vi "App - analyze RUS V6.vi"() -> ()   [LabVIEW 2018] (continued)
ry\\September_2014\\091614\\91.68500K_500_2500_2.10000V_0.00000T_Sep16-2014__23-15-32_001_091614.bin", "mod time(min)"=58229475.53333333, "file format"=enum."binary", "power(V)"=2.1, "Magn Field(T) "=0.0}, {"temperature"=91.557, "temperature str"="91.55700", "file path"=path "D:/Data/Ultrasound/LSCO/LSCO22__130814c/5_Cooling_2nd_try/September_2014/091614/91.55700K_500_2500_2.10000V_0.00000T_Sep16-2014__23-16-52_001_091614.bin", "last mod"=timestamp(3493768612 s since 1904-01-01), "file name str"="D:\\Data\\Ultrasound\\LSCO\\LSCO22__130814c\\5_Cooling_2nd_try\\September_2014\\091614\\91.55700K_500_2500_2.10000V_0.00000T_Sep16-2014__23-16-52_001_091614.bin", "mod time(min)"=58229476.86666667, "file format"=enum."binary", "power(V)"=2.1, "Magn Field(T) "=0.0}, {"temperature"=91.423, "temperature str"="91.42300", "file path"=path "D:/Data/Ultrasound/LSCO/LSCO22__130814c/5_Cooling_2nd_try/September_2014/091614/91.42300K_500_2500_2.10000V_0.00000T_Sep16-2014__23-18-11_001_091614.bin", "last mod"=timestamp(3493768691 s since 1904-01-01), "file name str"="D:\\Data\\Ultrasound\\LSCO\\LSCO22__130814c\\5_Cooling_2nd_try\\September_2014\\091614\\91.42300K_500_2500_2.10000V_0.00000T_Sep16-2014__23-18-11_001_091614.bin", "mod time(min)"=58229478.18333333, "file format"=enum."binary", "power(V)"=2.1, "Magn Field(T) "=0.0}, {"temperature"=91.291, "temperature str"="91.29100", "file path"=path "D:/Data/Ultrasound/LSCO/LSCO22__130814c/5_Cooling_2nd_try/September_2014/091614/91.29100K_500_2500_2.10000V_0.00000T_Sep16-2014__23-19-30_001_091614.bin", "last mod"=timestamp(3493768770 s since 1904-01-01), "file name str"="D:\\Data\\Ultrasound\\LSCO\\LSCO22__130814c\\5_Cooling_2nd_try\\September_2014\\091614\\91.29100K_500_2500_2.10000V_0.00000T_Sep16-2014__23-19-30_001_091614.bin", "mod time(min)"=58229479.5, "file format"=enum."binary", "power(V)"=2.1, "Magn Field(T) "=0.0}, {"temperature"=91.167, "temperature str"="91.16700", "file path"=path "D:/Data/Ultrasound/LSCO/LSCO22__130814c/5_Cooling_2nd_try/September_2014/091614/91.16700K_500_2500_2.10000V_0.00000T_Sep16-2014__23-20-50_001_091614.bin", "last mod"=timestamp(3493768850 s since 1904-01-01), "file name str"="D:\\Data\\Ultrasound\\LSCO\\LSCO22__130814c\\5_Cooling_2nd_try\\September_2014\\091614\\91.16700K_500_2500_2.10000V_0.00000T_Sep16-2014__23-20-50_001_091614.bin", "mod time(min)"=58229480.833333336, "file format"=enum."binary", "power(V)"=2.1, "Magn Field(T) "=0.0}, {"temperature"=91.035, "temperature str"="91.03500", "file path"=path "D:/Data/Ultrasound/LSCO/LSCO22__130814c/5_Cooling_2nd_try/September_2014/091614/91.03500K_500_2500_2.10000V_0.00000T_Sep16-2014__23-22-09_001_091614.bin", "last mod"=timestamp(3493768929 s since 1904-01-01), "file name str"="D:\\Data\\Ultrasound\\LSCO\\LSCO22__130814c\\5_Cooling_2nd_try\\September_2014\\091614\\91.03500K_500_2500_2.10000V_0.00000T_Sep16-2014__23-22-09_001_091614.bin", "mod time(min)"=58229482.15, "file format"=enum."binary", "power(V)"=2.1, "Magn Field(T) "=0.0}, {"temperature"=90.91, "temperature str"="90.91000", "file path"=path "D:/Data/Ultrasound/LSCO/LSCO22__130814c/5_Cooling_2nd_try/September_2014/091614/90.91000K_500_2500_2.10000V_0.00000T_Sep16-2014__23-23-28_001_091614.bin", "last mod"=timestamp(3493769008 s since 1904-01-01), "file name str"="D:\\Data\\Ultrasound\\LSCO\\LSCO22__130814c\\5_Cooling_2nd_try\\September_2014\\091614\\90.91000K_500_2500_2.10000V_0.00000T_Sep16-2014__23-23-28_001_091614.bin", "mod time(min)"=58229483.46666667, "file format"=enum."binary", "power(V)"=2.1, "Magn Field(T) "=0.0}, {"temperature"=90.778, "temperature str"="90.77800", "file path"=path "D:/Data/Ultrasound/LSCO/LSCO22__130814c/5_Cooling_2nd_try/September_2014/091614/90.77800K_500_2500_2.10000V_0.00000T_Sep16-2014__23-24-48_001_091614.bin", "last mod"=timestamp(3493769088 s since 1904-01-01), "file name str"="D:\\Data\\Ultrasound\\LSCO\\LSCO22__130814c\\5_Cooling_2nd_try\\September_2014\\091614\\90.77800K_500_2500_2.10000V_0.00000T_Sep16-2014__23-24-48_001_091614.bin", "mod time(min)"=58229484.8, "file format"=enum."binary", "power(V)"=2.1, "Magn Field(T) "=0.0}, {"temperature"=90.65, "temperature str"="90.65000", "file path"=path "D:/Data/Ultrasound/LSCO/LSCO22__130814c/5_Cooling_2nd_try/September_2014/091614/90.65000K_500_2500_2.10000V_0.00000T_Sep16-2014__23-26-07_001_091614.bin", "last mod"=timestamp(3493769167 s since 1904-01-01), "file name str"="D:\\Data\\Ultrasound\\LSCO\\LSCO22__130814c\\5_Cooling_2nd_try\\September_2014\\091614\\90.65000K_500_2500_2.10000V_0.00000T_Sep16-2014__23-26-07_001_091614.bin", "mod time(min)"=58229486.11666667, "file format"=enum."binary", "power(V)"=2.1, "Magn Field(T) "=0.0}, {"temperature"=90.526, "temperature str"="90.52600", "file path"=path "D:/Data/Ultrasound/LSCO/LSCO22__130814c/5_Cooling_2nd_try/September_2014/091614/90.52600K_500_2500_2.10000V_0.00000T_Sep16-2014__23-27-26_001_091614.bin", "last mod"=timestamp(3493769246 s since 1904-01-01), "file name str"="D:\\Data\\Ultrasound\\LSCO\\LSCO22__130814c\\5_Cooling_2nd_try\\September_2014\\091614\\90.52600K_500_2500_2.10000V_0.00000T_Sep16-2014__23-27-26_001_091614.bin", "mod time(min)"=58229487.43333333, "file format"=enum."binary", "power(V)"=2.1, "Magn Field(T) "=0.0}, {"temperature"=90.397, "temperature str"="90.39700", "file path"=path "D:/Data/Ultrasound/LSCO/LSCO22__130814c/5_Cooling_2nd_try/September_2014/091614/90.39700K_500_2500_2.10000V_0.00000T_Sep16-2014__23-28-46_001_091614.bin", "last mod"=timestamp(3493769326 s since 1904-01-01), "file name str"="D:\\Data\\Ultrasound\\LSCO\\LSCO22__130814c\\5_Cooling_2nd_try\\September_2014\\091614\\90.39700K_500_2500_2.10000V_0.00000T_Sep16-2014__23-28-46_001_091614.bin", "mod time(min)"=58229488.766666666, "file format"=enum."binary", "power(V)"=2.1, "Magn Field(T) "=0.0}, {"temperature"=90.276, "temperature str"="90.27600", "file path"=path "D:/Data/Ultrasound/LSCO/LSCO22__130814c/5_Cooling_2nd_try/September_2014/091614/90.27600K_500_2500_2.10000V_0.00000T_Sep16-2014__23-30-05_001_091614.bin", "last mod"=timestamp(3493769405 s since 1904-01-01), "file name str"="D:\\Data\\Ultrasound\\LSCO\\LSCO22__130814c\\5_Cooling_2nd_try\\September_2014\\091614\\90.27600K_500_2500_2.10000V_0.00000T_Sep16-2014__23-30-05_001_091614.bin", "mod time(min)"=58229490.083333336, "file format"=enum."binary", "power(V)"=2.1, "Magn Field(T) "=0.0}, {"temperature"=90.146, "temperature str"="90.14600", "file path"=path "D:/Data/Ultrasound/LSCO/LSCO22__130814c/5_Cooling_2nd_try/September_2014/091614/90.14600K_500_2500_2.10000V_0.00000T_Sep16-2014__23-31-25_001_091614.bin", "last mod"=timestamp(3493769485 s since 1904-01-01), "file name str"="D:\\Data\\Ultrasound\\LSCO\\LSCO22__130814c\\5_Cooling_2nd_try\\September_2014\\091614\\90.14600K_500_2500_2.10000V_0.00000T_Sep16-2014__23-31-25_001_091614.bin", "mod time(min)"=58229491.416666664, "file format"=enum."binary", "power(V)"=2.1, "Magn Field(T) "=0.0}, {"temperature"=90.022, "temperature str"="90.02200", "file path"=path "D:/Data/Ultrasound/LSCO/LSCO22__130814c/5_Cooling_2nd_try/September_2014/091614/90.02200K_500_2500_2.10000V_0.00000T_Sep16-2014__23-32-44_001_091614.bin", "last mod"=timestamp(3493769564 s since 1904-01-01), "file name str"="D:\\Data\\Ultrasound\\LSCO\\LSCO22__130814c\\5_Cooling_2nd_try\\September_2014\\091614\\90.02200K_500_2500_2.10000V_0.00000T_Sep16-2014__23-32-44_001_091614.bin", "mod time(min)"=58229492.733333334, "file format"=enum."binary", "power(V)"=2.1, "Magn Field(T) "=0.0}, {"temperature"=89.9, "temperature str"="89.90000", "file path"=path "D:/Data/Ultrasound/LSCO/LSCO22__130814c/5_Cooling_2nd_try/September_2014/091614/89.90000K_500_2500_2.10000V_0.00000T_Sep16-2014__23-34-03_001_091614.bin", "last mod"=timestamp(3493769643 s since 1904-01-01), "file name str"="D:\\Data\\Ultrasound\\LSCO\\LSCO22__130814c\\5_Cooling_2nd_try\\September_2014\\091614\\89.90000K_500_2500_2.10000V_0.00000T_Sep16-2014__23-34-03_001_091614.bin", "mod time(min)"=58229494.05, "file format"=enum."binary", "power(V)"=2.1, "Magn Field(T) "=0.0}, {"temperature"=89.775, "temperature str"="89.77500", "file path"=path "D:/Data/Ultrasound/LSCO/LSCO22__130814c/5_Cooling_2nd_try/September_2014/091614/89.77500K_500_2500_2.10000V_0.00000T_Sep16-2014__23-35-23_001_091614.bin", "last mod"=timestamp(3493769723 s since 1904-01-01), "file name str"="D:\\Data\\Ultrasound\\LSCO\\LSCO22__130814c\\5_Cooling_2nd_try\\September_2014\\091614\\89.77500K_500_2500_2.10000V_0.00000T_Sep16-2014__23-35-23_001_091614.bin", "mod time(min)"=58229495.38333333, "file format"=enum."binary", "power(V)"=2.1, "Magn Field(T) "=0.0}, {"temperature"=89.652, "temperature str"="89.65200", "file path"=path "D:/Data/Ultrasound/LSCO/LSCO22__130814c/5_Cooling_2nd_try/September_2014/091614/89.65200K_500_2500_2.10000V_0.00000T_Sep16-2014__23-36-42_001_091614.bin", "last mod"=timestamp(3493769802 s since 1904-01-01), "file name str"="D:\\Data\\Ultrasound\\LSCO\\LSCO22__130814c\\5_Cooling_2nd_try\\September_2014\\091614\\89.65200K_500_2500_2.10000V_0.00000T_Sep16-2014__23-36-42_001_091614.bin", "mod time(min)"=58229496.7, "file format"=enum."binary", "power(V)"=2.1, "Magn Field(T) "=0.0}, {"temperature"=89.531, "temperature str"="89.53100", "file path"=path "D:/Data/Ultrasound/LSCO/LSCO22__130814c/5_Cooling_2nd_try/September_2014/091614/89.53100K_500_2500_2.10000V_0.00000T_Sep16-2014__23-38-01_001_091614.bin", "last mod"=timestamp(3493769881 s since 1904-01-01), "file name str"="D:\\Data\\Ultrasound\\LSCO\\LSCO22__130814c\\5_Cooling_2nd_try\\September_2014\\091614\\89.53100K_500_2500_2.10000V_0.00000T_Sep16-2014__23-38-01_001_091614.bin", "mod time(min)"=58229498.016666666, "file format"=enum."binary", "power(V)"=2.1, "Magn Field(T) "=0.0}, {"temperature"=89.405, "temperature str"="89.40500", "file path"=path "D:/Data/Ultrasound/LSCO/LSCO22__130814c/5_Cooling_2nd_try/September_2014/091614/89.40500K_500_2500_2.10000V_0.00000T_Sep16-2014__23-39-21_001_091614.bin", "last mod"=timestamp(3493769961 s since 1904-01-01), "file name str"="D:\\Data\\Ultrasound\\LSCO\\LSCO22__130814c\\5_Cooling_2nd_try\\September_2014\\091614\\89.40500K_500_2500_2.10000V_0.00000T_Sep16-2014__23-39-21_001_091614.bin", "mod time(min)"=58229499.35, "file format"=enum."binary", "power(V)"=2.1, "Magn Field(T) "=0.0}, {"temperature"=89.288, "temperature str"="89.28800", "file path"=path "D:/Data/Ultrasound/LSCO/LSCO22__130814c/5_Cooling_2nd_try/September_2014/091614/89.28800K_500_2500_2.10000V_0.00000T_Sep16-2014__23-40-40_001_091614.bin", "last mod"=timestamp(3493770040 s since 1904-01-01), "file name str"="D:\\Data\\Ultrasound\\LSCO\\LSCO22__130814c\\5_Cooling_2nd_try\\September_2014\\091614\\89.28800K_500_2500_2.10000V_0.00000T_Sep16-2014__23-40-40_001_091614.bin", "mod time(min)"=58229500.666666664, "file format"=enum."binary", "power(V)"=2.1, "Magn Field(T) "=0.0}, {"temperature"=89.165, "temperature str"="89.16500", "file path"=path "D:/Data/Ultrasound/LSCO/LSCO22__130814c/5_Cooling_2nd_try/September_2014/091614/89.16500K_500_2500_2.10000V_0.00000T_Sep16-2014__23-42-00_001_091614.bin", "last mod"=timestamp(3493770120 s since 1904-01-01), "file name str"="D:\\Data\\Ultrasound\\LSCO\\LSCO22__130814c\\5_Cooling_2nd_try\\September_2014\\091614\\89.16500K_500_2500_2.10000V_0.00000T_Sep16-2014__23-42-00_001_091614.bin", "mod time(min)"=58229502.0, "file format"=enum."binary", "power(V)"=2.1, "Magn Field(T) "=0.0}, {"temperature"=89.042, "temperature str"="89.04200", "file path"=path "D:/Data/Ultrasound/LSCO/LSCO22__130814c/5_Cooling_2nd_try/September_2014/091614/89.04200K_500_2500_2.10000V_0.00000T_Sep16-2014__23-43-19_001_091614.bin", "last mod"=timestamp(3493770199 s since 1904-01-01), "file name str"="D:\\Data\\Ultrasound\\LSCO\\LSCO22__130814c\\5_Cooling_2nd_try\\September_2014\\091614\\89.04200K_500_2500_2.10000V_0.00000T_Sep16-2014__23-43-19_001_091614.bin", "mod time(min)"=58229503.31666667, "file format"=enum."binary", "power(V)"=2.1, "Magn Field(T) "=0.0}, {"temperature"=88.925, "temperature str"="88.92500", "file path"=path "D:/Data/Ultrasound/LSCO/LSCO22__130814c/5_Cooling_2nd_try/September_2014/091614/88.92500K_500_2500_2.10000V_0.00000T_Sep16-2014__23-44-38_001_091614.bin", "last mod"=timestamp(3493770278 s since 1904-01-01), "file name str"="D:\\Data\\Ultrasound\\LSCO\\LSCO22__130814c\\5_Cooling_2nd_try\\September_2014\\091614\\88.92500K_500_2500_2.10000V_0.00000T_Sep16-2014__23-44-38_001_091614.bin", "mod time(min)"=58229504.63333333, "file format"=enum."binary", "power(V)"=2.1, "Magn Field(T) "=0.0}, {"temperature"=88.804, "temperature str"="88.80400", "file path"=path "D:/Data/Ultrasound/LSCO/LSCO22__130814c/5_Cooling_2nd_try/September_2014/091614/88.80400K_500_2500_2.10000V_0.00000T_Sep16-2014__23-45-58_001_091614.bin", "last mod"=timestamp(3493770358 s since 1904-01-01), "file name str"="D:\\Data\\Ultrasound\\LSCO\\LSCO22__130814c\\5_Cooling_2nd_try\\September_2014\\091614\\88.80400K_500_2500_2.10000V_0.00000T_Sep16-2014__23-45-58_001_091614.bin", "mod time(min)"=58229505.96666667, "file format"=enum."binary", "power(V)"=2.1, "Magn Field(T) "=0.0}, {"temperature"=88.687, "temperature str"="88.68700", "file path"=path "D:/Data/Ultrasound/LSCO/LSCO22__130814c/5_Cooling_2nd_try/September_2014/091614/88.68700K_500_2500_2.10000V_0.00000T_Sep16-2014__23-47-17_001_091614.bin", "last mod"=timestamp(3493770437 s since 1904-01-01), "file name str"="D:\\Data\\Ultrasound\\LSCO\\LSCO22__130814c\\5_Cooling_2nd_try\\September_2014\\091614\\88.68700K_500_2500_2.10000V_0.00000T_Sep16-2014__23-47-17_001_091614.bin", "mod time(min)"=58229507.28333333, "file format"=enum."binary", "power(V)"=2.1, "Magn Field(T) "=0.0}, {"temperature"=88.566, "temperature str"="88.56600", "file path"=path "D:/Data/Ultrasound/LSCO/LSCO22__130814c/5_Cooling_2nd_try/September_2014/091614/88.56600K_500_2500_2.10000V_0.00000T_Sep16-2014__23-48-36_001_091614.bin", "last mod"=timestamp(3493770516 s since 1904-01-01), "file name str"="D:\\Data\\Ultrasound\\LSCO\\LSCO22__130814c\\5_Cooling_2nd_try\\September_2014\\091614\\88.56600K_500_2500_2.10000V_0.00000T_Sep16-2014__23-48-36_001_091614.bin", "mod time(min)"=58229508.6, "file format"=enum."binary", "power(V)"=2.1, "Magn Field(T) "=0.0}, {"temperature"=88.447, "temperature str"="88.44700", "file path"=path "D:/Data/Ultrasound/LSCO/LSCO22__130814c/5_Cooling_2nd_try/September_2014/091614/88.44700K_500_2500_2.10000V_0.00000T_Sep16-2014__23-49-56_001_091614.bin", "last mod"=timestamp(3493770596 s since 1904-01-01), "file name str"="D:\\Data\\Ultrasound\\LSCO\\LSCO22__130814c\\5_Cooling_2nd_try\\September_2014\\091614\\88.44700K_500_2500_2.10000V_0.00000T_Sep16-2014__23-49-56_001_091614.bin", "mod time(min)"=58229509.93333333, "file format"=enum."binary", "power(V)"=2.1, "Magn Field(T) "=0.0}, {"temperature"=88.332, "temperature str"="88.33200", "file path"=path "D:/Data/Ultrasound/LSCO/LSCO22__130814c/5_Cooling_2nd_try/September_2014/091614/88.33200K_500_2500_2.10000V_0.00000T_Sep16-2014__23-51-15_001_091614.bin", "last mod"=timestamp(3493770675 s since 1904-01-01), "file name str"="D:\\Data\\Ultrasound\\LSCO\\LSCO22__130814c\\5_Cooling_2nd_try\\September_2014\\091614\\88.33200K_500_2500_2.10000V_0.00000T_Sep16-2014__23-51-15_001_091614.bin", "mod time(min)"=58229511.25, "file format"=enum."binary", "power(V)"=2.1, "Magn Field(T) "=0.0}, {"temperature"=88.213, "temperature str"="88.21300", "file path"=path "D:/Data/Ultrasound/LSCO/LSCO22__130814c/5_Cooling_2nd_try/September_2014/091614/88.21300K_500_2500_2.10000V_0.00000T_Sep16-2014__23-52-35_001_091614.bin", "last mod"=timestamp(3493770755 s since 1904-01-01), "file name str"="D:\\Data\\Ultrasound\\LSCO\\LSCO22__130814c\\5_Cooling_2nd_try\\September_2014\\091614\\88.21300K_500_2500_2.10000V_0.00000T_Sep16-2014__23-52-35_001_091614.bin", "mod time(min)"=58229512.583333336, "file format"=enum."binary", "power(V)"=2.1, "Magn Field(T) "=0.0}, {"temperature"=88.1, "temperature str"="88.10000", "file path"=path "D:/Data/Ultrasound/LSCO/LSCO22__130814c/5_Cooling_2nd_try/September_2014/091614/88.10000K_500_2500_2.10000V_0.00000T_Sep16-2014__23-53-54_001_091614.bin", "last mod"=timestamp(3493770834 s since 1904-01-01), "file name str"="D:\\Data\\Ultrasound\\LSCO\\LSCO22__130814c\\5_Cooling_2nd_try\\September_2014\\091614\\88.10000K_500_2500_2.10000V_0.00000T_Sep16-2014__23-53-54_001_091614.bin", "mod time(min)"=58229513.9, "file format"=enum."binary", "power(V)"=2.1, "Magn Field(T) "=0.0}, {"temperature"=87.983, "temperature str"="87.98300", "file path"=path "D:/Data/Ultrasound/LSCO/LSCO22__130814c/5_Cooling_2nd_try/September_2014/091614/87.98300K_500_2500_2.10000V_0.00000T_Sep16-2014__23-55-13_001_091614.bin", "last mod"=timestamp(3493770913 s since 1904-01-01), "file name str"="D:\\Data\\Ultrasound\\LSCO\\LSCO22__130814c\\5_Cooling_2nd_try\\September_2014\\091614\\87.98300K_500_2500_2.10000V_0.00000T_Sep16-2014__23-55-13_001_091614.bin", "mod time(min)"=58229515.21666667, "file format"=enum."binary", "power(V)"=2.1, "Magn Field(T) "=0.0}, {"temperature"=87.861, "temperature str"="87.86100", "file path"=path "D:/Data/Ultrasound/LSCO/LSCO22__130814c/5_Cooling_2nd_try/September_2014/091614/87.86100K_500_2500_2.10000V_0.00000T_Sep16-2014__23-56-33_001_091614.bin", "last mod"=timestamp(3493770993 s since 1904-01-01), "file name str"="D:\\Data\\Ultrasound\\LSCO\\LSCO22__130814c\\5_Cooling_2nd_try\\September_2014\\091614\\87.86100K_500_2500_2.10000V_0.00000T_Sep16-2014__23-56-33_001_091614.bin", "mod time(min)"=58229516.55, "file format"=enum."binary", "power(V)"=2.1, "Magn Field(T) "=0.0}, {"temperature"=87.751, "temperature str"="87.75100", "file path"=path "D:/Data/Ultrasound/LSCO/LSCO22__130814c/5_Cooling_2nd_try/September_2014/091614/87.75100K_500_2500_2.10000V_0.00000T_Sep16-2014__23-57-52_001_091614.bin", "last mod"=timestamp(3493771072 s since 1904-01-01), "file name str"="D:\\Data\\Ultrasound\\LSCO\\LSCO22__130814c\\5_Cooling_2nd_try\\September_2014\\091614\\87.75100K_500_2500_2.10000V_0.00000T_Sep16-2014__23-57-52_001_091614.bin", "mod time(min)"=58229517.86666667, "file format"=enum."binary", "power(V)"=2.1, "Magn Field(T) "=0.0}, {"temperature"=87.635, "temperature str"="87.63500", "file path"=path "D:/Data/Ultrasound/LSCO/LSCO22__130814c/5_Cooling_2nd_try/September_2014/091714/87.63500K_500_2500_2.10000V_0.00000T_Sep16-2014__23-59-11_001_091714.bin", "last mod"=timestamp(3493771151 s since 1904-01-01), "file name str"="D:\\Data\\Ultrasound\\LSCO\\LSCO22__130814c\\5_Cooling_2nd_try\\September_2014\\091714\\87.63500K_500_2500_2.10000V_0.00000T_Sep16-2014__23-59-11_001_091714.bin", "mod time(min)"=58229519.18333333, "file format"=enum."binary", "power(V)"=2.1, "Magn Field(T) "=0.0}, {"temperature"=87.523, "temperature str"="87.52300", "file path"=path "D:/Data/Ultrasound/LSCO/LSCO22__130814c/5_Cooling_2nd_try/September_2014/091714/87.52300K_500_2500_2.10000V_0.00000T_Sep17-2014__00-00-31_001_091714.bin", "last mod"=timestamp(3493771231 s since 1904-01-01), "file name str"="D:\\Data\\Ultrasound\\LSCO\\LSCO22__130814c\\5_Cooling_2nd_try\\September_2014\\091714\\87.52300K_500_2500_2.10000V_0.00000T_Sep17-2014__00-00-31_001_091714.bin", "mod time(min)"=58229520.516666666, "file format"=enum."binary", "power(V)"=2.1, "Magn Field(T) "=0.0}, {"temperature"=87.407, "temperature str"="87.40700", "file path"=path "D:/Data/Ultrasound/LSCO/LSCO22__130814c/5_Cooling_2nd_try/September_2014/091714/87.40700K_500_2500_2.10000V_0.00000T_Sep17-2014__00-01-50_001_091714.bin", "last mod"=timestamp(3493771310 s since 1904-01-01), "file name str"="D:\\Data\\Ultrasound\\LSCO\\LSCO22__130814c\\5_Cooling_2nd_try\\September_2014\\091714\\87.40700K_500_2500_2.10000V_0.00000T_Sep17-2014__00-01-50_001_091714.bin", "mod time(min)"=58229521.833333336, "file format"=enum."binary", "power(V)"=2.1, "Magn Field(T) "=0.0}, {"temperature"=87.293, "temperature str"="87.29300", "file path"=path "D:/Data/Ultrasound/LSCO/LSCO22__130814c/5_Cooling_2nd_try/September_2014/091714/87.29300K_500_2500_2.10000V_0.00000T_Sep17-2014__00-03-10_001_091714.bin", "last mod"=timestamp(3493771390 s since 1904-01-01), "file name str"="D:\\Data\\Ultrasound\\LSCO\\LSCO22__130814c\\5_Cooling_2nd_try\\September_2014\\091714\\87.29300K_500_2500_2.10000V_0.00000T_Sep17-2014__00-03-10_001_091714.bin", "mod time(min)"=58229523.166666664, "file format"=enum."binary", "power(V)"=2.1, "Magn Field(T) "=0.0}, {"temperature"=87.182, "temperature str"="87.18200", "file path"=path "D:/Data/Ultrasound/LSCO/LSCO22__130814c/5_Cooling_2nd_try/September_2014/091714/87.18200K_500_2500_2.10000V_0.00000T_Sep17-2014__00-04-29_001_091714.bin", "last mod"=timestamp(3493771469 s since 1904-01-01), "file name str"="D:\\Data\\Ultrasound\\LSCO\\LSCO22__130814c\\5_Cooling_2nd_try\\September_2014\\091714\\87.18200K_500_2500_2.10000V_0.00000T_Sep17-2014__00-04-29_001_091714.bin", "mod time(min)"=58229524.483333334, "file format"=enum."binary", "power(V)"=2.1, "Magn Field(T) "=0.0}, {"temperature"=87.068, "temperature str"="87.06800", "file path"=path "D:/Data/Ultrasound/LSCO/LSCO22__130814c/5_Cooling_2nd_try/September_2014/091714/87.06800K_500_2500_2.10000V_0.00000T_Sep17-2014__00-05-48_001_091714.bin", "last mod"=timestamp(3493771548 s since 1904-01-01), "file name str"="D:\\Data\\Ultrasound\\LSCO\\LSCO22__130814c\\5_Cooling_2nd_try\\September_2014\\091714\\87.06800K_500_2500_2.10000V_0.00000T_Sep17-2014__00-05-48_001_091714.bin", "mod time(min)"=58229525.8, "file format"=enum."binary", "power(V)"=2.1, "Magn Field(T) "=0.0}, {"temperature"=86.958, "temperature str"="86.95800", "file path"=path "D:/Data/Ultrasound/LSCO/LSCO22__130814c/5_Cooling_2nd_try/September_2014/091714/86.95800K_500_2500_2.10000V_0.00000T_Sep17-2014__00-07-08_001_091714.bin", "last mod"=timestamp(3493771628 s since 1904-01-01), "file name str"="D:\\Data\\Ultrasound\\LSCO\\LSCO22__130814c\\5_Cooling_2nd_try\\September_2014\\091714\\86.95800K_500_2500_2.10000V_0.00000T_Sep17-2014__00-07-08_001_091714.bin", "mod time(min)"=58229527.13333333, "file format"=enum."binary", "power(V)"=2.1, "Magn Field(T) "=0.0}, {"temperature"=86.845, "temperature str"="86.84500", "file path"=path "D:/Data/Ultrasound/LSCO/LSCO22__130814c/5_Cooling_2nd_try/September_2014/091714/86.84500K_500_2500_2.10000V_0.00000T_Sep17-2014__00-08-27_001_091714.bin", "last mod"=timestamp(3493771707 s since 1904-01-01), "file name str"="D:\\Data\\Ultrasound\\LSCO\\LSCO22__130814c\\5_Cooling_2nd_try\\September_2014\\091714\\86.84500K_500_2500_2.10000V_0.00000T_Sep17-2014__00-08-27_001_091714.bin", "mod time(min)"=58229528.45, "file format"=enum."binary", "power(V)"=2.1, "Magn Field(T) "=0.0}, {"temperature"=86.732, "temperature str"="86.73200", "file path"=path "D:/Data/Ultrasound/LSCO/LSCO22__130814c/5_Cooling_2nd_try/September_2014/091714/86.73200K_500_2500_2.10000V_0.00000T_Sep17-2014__00-09-46_001_091714.bin", "last mod"=timestamp(3493771786 s since 1904-01-01), "file name str"="D:\\Data\\Ultrasound\\LSCO\\LSCO22__130814c\\5_Cooling_2nd_try\\September_2014\\091714\\86.73200K_500_2500_2.10000V_0.00000T_Sep17-2014__00-09-46_001_091714.bin", "mod time(min)"=58229529.766666666, "file format"=enum."binary", "power(V)"=2.1, "Magn Field(T) "=0.0}, {"temperature"=86.623, "temperature str"="86.62300", "file path"=path "D:/Data/Ultrasound/LSCO/LSCO22__130814c/5_Cooling_2nd_try/September_2014/091714/86.62300K_500_2500_2.10000V_0.00000T_Sep17-2014__00-11-06_001_091714.bin", "last mod"=timestamp(3493771866 s since 1904-01-01), "file name str"="D:\\Data\\Ultrasound\\LSCO\\LSCO22__130814c\\5_Cooling_2nd_try\\September_2014\\091714\\86.62300K_500_2500_2.10000V_0.00000T_Sep17-2014__00-11-06_001_091714.bin", "mod time(min)"=58229531.1, "file format"=enum."binary", "power(V)"=2.1, "Magn Field(T) "=0.0}, {"temperature"=86.512, "temperature str"="86.51200", "file path"=path "D:/Data/Ultrasound/LSCO/LSCO22__130814c/5_Cooling_2nd_try/September_2014/091714/86.51200K_500_2500_2.10000V_0.00000T_Sep17-2014__00-12-25_001_091714.bin", "last mod"=timestamp(3493771945 s since 1904-01-01), "file name str"="D:\\Data\\Ultrasound\\LSCO\\LSCO22__130814c\\5_Cooling_2nd_try\\September_2014\\091714\\86.51200K_500_2500_2.10000V_0.00000T_Sep17-2014__00-12-25_001_091714.bin", "mod time(min)"=58229532.416666664, "file format"=enum."binary", "power(V)"=2.1, "Magn Field(T) "=0.0}, {"temperature"=86.405, "temperature str"="86.40500", "file path"=path "D:/Data/Ultrasound/LSCO/LSCO22__130814c/5_Cooling_2nd_try/September_2014/091714/86.40500K_500_2500_2.10000V_0.00000T_Sep17-2014__00-13-45_001_091714.bin", "last mod"=timestamp(3493772025 s since 1904-01-01), "file name str"="D:\\Data\\Ultrasound\\LSCO\\LSCO22__130814c\\5_Cooling_2nd_try\\September_2014\\091714\\86.40500K_500_2500_2.10000V_0.00000T_Sep17-2014__00-13-45_001_091714.bin", "mod time(min)"=58229533.75, "file format"=enum."binary", "power(V)"=2.1, "Magn Field(T) "=0.0}, {"temperature"=86.294, "temperature str"="86.29400", "file path"=path "D:/Data/Ultrasound/LSCO/LSCO22__130814c/5_Cooling_2nd_try/September_2014/091714/86.29400K_500_2500_2.10000V_0.00000T_Sep17-2014__00-15-04_001_091714.bin", "last mod"=timestamp(3493772104 s since 1904-01-01), "file name str"="D:\\Data\\Ultrasound\\LSCO\\LSCO22__130814c\\5_Cooling_2nd_try\\September_2014\\091714\\86.29400K_500_2500_2.10000V_0.00000T_Sep17-2014__00-15-04_001_091714.bin", "mod time(min)"=58229535.06666667, "file format"=enum."binary", "power(V)"=2.1, "Magn Field(T) "=0.0}, {"temperature"=86.184, "temperature str"="86.18400", "file path"=path "D:/Data/Ultrasound/LSCO/LSCO22__130814c/5_Cooling_2nd_try/September_2014/091714/86.18400K_500_2500_2.10000V_0.00000T_Sep17-2014__00-16-23_001_091714.bin", "last mod"=timestamp(3493772183 s since 1904-01-01), "file name str"="D:\\Data\\Ultrasound\\LSCO\\LSCO22__130814c\\5_Cooling_2nd_try\\September_2014\\091714\\86.18400K_500_2500_2.10000V_0.00000T_Sep17-2014__00-16-23_001_091714.bin", "mod time(min)"=58229536.38333333, "file format"=enum."binary", "power(V)"=2.1, "Magn Field(T) "=0.0}, {"temperature"=86.077, "temperature str"="86.07700", "file path"=path "D:/Data/Ultrasound/LSCO/LSCO22__130814c/5_Cooling_2nd_try/September_2014/091714/86.07700K_500_2500_2.10000V_0.00000T_Sep17-2014__00-17-43_001_091714.bin", "last mod"=timestamp(3493772263 s since 1904-01-01), "file name str"="D:\\Data\\Ultrasound\\LSCO\\LSCO22__130814c\\5_Cooling_2nd_try\\September_2014\\091714\\86.07700K_500_2500_2.10000V_0.00000T_Sep17-2014__00-17-43_001_091714.bin", "mod time(min)"=58229537.71666667, "file format"=enum."binary", "power(V)"=2.1, "Magn Field(T) "=0.0}, {"temperature"=85.969, "temperature str"="85.96900", "file path"=path "D:/Data/Ultrasound/LSCO/LSCO22__130814c/5_Cooling_2nd_try/September_2014/091714/85.96900K_500_2500_2.10000V_0.00000T_Sep17-2014__00-19-02_001_091714.bin", "last mod"=timestamp(3493772342 s since 1904-01-01), "file name str"="D:\\Data\\Ultrasound\\LSCO\\LSCO22__130814c\\5_Cooling_2nd_try\\September_2014\\091714\\85.96900K_500_2500_2.10000V_0.00000T_Sep17-2014__00-19-02_001_091714.bin", "mod time(min)"=58229539.03333333, "file format"=enum."binary", "power(V)"=2.1, "Magn Field(T) "=0.0}, {"temperature"=85.861, "temperature str"="85.86100", "file path"=path "D:/Data/Ultrasound/LSCO/LSCO22__130814c/5_Cooling_2nd_try/September_2014/091714/85.86100K_500_2500_2.10000V_0.00000T_Sep17-2014__00-20-21_001_091714.bin", "last mod"=timestamp(3493772421 s since 1904-01-01), "file name str"="D:\\Data\\Ultrasound\\LSCO\\LSCO22__130814c\\5_Cooling_2nd_try\\September_2014\\091714\\85.86100K_500_2500_2.10000V_0.00000T_Sep17-2014__00-20-21_001_091714.bin", "mod time(min)"=58229540.35, "file format"=enum."binary", "power(V)"=2.1, "Magn Field(T) "=0.0}, {"temperature"=85.752, "temperature str"="85.75200", "file path"=path "D:/Data/Ultrasound/LSCO/LSCO22__130814c/5_Cooling_2nd_try/September_2014/091714/85.75200K_500_2500_2.10000V_0.00000T_Sep17-2014__00-21-41_001_091714.bin", "last mod"=timestamp(3493772501 s since 1904-01-01), "file name str"="D:\\Data\\Ultrasound\\LSCO\\LSCO22__130814c\\5_Cooling_2nd_try\\September_2014\\091714\\85.75200K_500_2500_2.10000V_0.00000T_Sep17-2014__00-21-41_001_091714.bin", "mod time(min)"=58229541.68333333, "file format"=enum."binary", "power(V)"=2.1, "Magn Field(T) "=0.0}, {"temperature"=85.645, "temperature str"="85.64500", "file path"=path "D:/Data/Ultrasound/LSCO/LSCO22__130814c/5_Cooling_2nd_try/September_2014/091714/85.64500K_500_2500_2.10000V_0.00000T_Sep17-2014__00-23-00_001_091714.bin", "last mod"=timestamp(3493772580 s since 1904-01-01), "file name str"="D:\\Data\\Ultrasound\\LSCO\\LSCO22__130814c\\5_Cooling_2nd_try\\September_2014\\091714\\85.64500K_500_2500_2.10000V_0.00000T_Sep17-2014__00-23-00_001_091714.bin", "mod time(min)"=58229543.0, "file format"=enum."binary", "power(V)"=2.1, "Magn Field(T) "=0.0}, {"temperature"=85.541, "temperature str"="85.54100", "file path"=path "D:/Data/Ultrasound/LSCO/LSCO22__130814c/5_Cooling_2nd_try/September_2014/091714/85.54100K_500_2500_2.10000V_0.00000T_Sep17-2014__00-24-20_001_091714.bin", "last mod"=timestamp(3493772660 s since 1904-01-01), "file name str"="D:\\Data\\Ultrasound\\LSCO\\LSCO22__130814c\\5_Cooling_2nd_try\\September_2014\\091714\\85.54100K_500_2500_2.10000V_0.00000T_Sep17-2014__00-24-20_001_091714.bin", "mod time(min)"=58229544.333333336, "file format"=enum."binary", "power(V)"=2.1, "Magn Field(T) "=0.0}, {"temperature"=85.433, "temperature str"="85.43300", "file path"=path "D:/Data/Ultrasound/LSCO/LSCO22__130814c/5_Cooling_2nd_try/September_2014/091714/85.43300K_500_2500_2.10000V_0.00000T_Sep17-2014__00-25-39_001_091714.bin", "last mod"=timestamp(3493772739 s since 1904-01-01), "file name str"="D:\\Data\\Ultrasound\\LSCO\\LSCO22__130814c\\5_Cooling_2nd_try\\September_2014\\091714\\85.43300K_500_2500_2.10000V_0.00000T_Sep17-2014__00-25-39_001_091714.bin", "mod time(min)"=58229545.65, "file format"=enum."binary", "power(V)"=2.1, "Magn Field(T) "=0.0}, {"temperature"=85.328, "temperature str"="85.32800", "file path"=path "D:/Data/Ultrasound/LSCO/LSCO22__130814c/5_Cooling_2nd_try/September_2014/091714/85.32800K_500_2500_2.10000V_0.00000T_Sep17-2014__00-26-58_001_091714.bin", "last mod"=timestamp(3493772818 s since 1904-01-01), "file name str"="D:\\Data\\Ultrasound\\LSCO\\LSCO22__130814c\\5_Cooling_2nd_try\\September_2014\\091714\\85.32800K_500_2500_2.10000V_0.00000T_Sep17-2014__00-26-58_001_091714.bin", "mod time(min)"=58229546.96666667, "file format"=enum."binary", "power(V)"=2.1, "Magn Field(T) "=0.0}, {"temperature"=85.224, "temperature str"="85.22400", "file path"=path "D:/Data/Ultrasound/LSCO/LSCO22__130814c/5_Cooling_2nd_try/September_2014/091714/85.22400K_500_2500_2.10000V_0.00000T_Sep17-2014__00-28-18_001_091714.bin", "last mod"=timestamp(3493772898 s since 1904-01-01), "file name str"="D:\\Data\\Ultrasound\\LSCO\\LSCO22__130814c\\5_Cooling_2nd_try\\September_2014\\091714\\85.22400K_500_2500_2.10000V_0.00000T_Sep17-2014__00-28-18_001_091714.bin", "mod time(min)"=58229548.3, "file format"=enum."binary", "power(V)"=2.1, "Magn Field(T) "=0.0}, {"temperature"=85.117, "temperature str"="85.11700", "file path"=path "D:/Data/Ultrasound/LSCO/LSCO22__130814c/5_Cooling_2nd_try/September_2014/091714/85.11700K_500_2500_2.10000V_0.00000T_Sep17-2014__00-29-37_001_091714.bin", "last mod"=timestamp(3493772977 s since 1904-01-01), "file name str"="D:\\Data\\Ultrasound\\LSCO\\LSCO22__130814c\\5_Cooling_2nd_try\\September_2014\\091714\\85.11700K_500_2500_2.10000V_0.00000T_Sep17-2014__00-29-37_001_091714.bin", "mod time(min)"=58229549.61666667, "file format"=enum."binary", "power(V)"=2.1, "Magn Field(T) "=0.0}, {"temperature"=85.014, "temperature str"="85.01400", "file path"=path "D:/Data/Ultrasound/LSCO/LSCO22__130814c/5_Cooling_2nd_try/September_2014/091714/85.01400K_500_2500_2.10000V_0.00000T_Sep17-2014__00-30-56_001_091714.bin", "last mod"=timestamp(3493773056 s since 1904-01-01), "file name str"="D:\\Data\\Ultrasound\\LSCO\\LSCO22__130814c\\5_Cooling_2nd_try\\September_2014\\091714\\85.01400K_500_2500_2.10000V_0.00000T_Sep17-2014__00-30-56_001_091714.bin", "mod time(min)"=58229550.93333333, "file format"=enum."binary", "power(V)"=2.1, "Magn Field(T) "=0.0}, {"temperature"=84.907, "temperature str"="84.90700", "file path"=path "D:/Data/Ultrasound/LSCO/LSCO22__130814c/5_Cooling_2nd_try/September_2014/091714/84.90700K_500_2500_2.10000V_0.00000T_Sep17-2014__00-32-16_001_091714.bin", "last mod"=timestamp(3493773136 s since 1904-01-01), "file name str"="D:\\Data\\Ultrasound\\LSCO\\LSCO22__130814c\\5_Cooling_2nd_try\\September_2014\\091714\\84.90700K_500_2500_2.10000V_0.00000T_Sep17-2014__00-32-16_001_091714.bin", "mod time(min)"=58229552.266666666, "file format"=enum."binary", "power(V)"=2.1, "Magn Field(T) "=0.0}, {"temperature"=84.805, "temperature str"="84.80500", "file path"=path "D:/Data/Ultrasound/LSCO/LSCO22__130814c/5_Cooling_2nd_try/September_2014/091714/84.80500K_500_2500_2.10000V_0.00000T_Sep17-2014__00-33-35_001_091714.bin", "last mod"=timestamp(3493773215 s since 1904-01-01), "file name str"="D:\\Data\\Ultrasound\\LSCO\\LSCO22__130814c\\5_Cooling_2nd_try\\September_2014\\091714\\84.80500K_500_2500_2.10000V_0.00000T_Sep17-2014__00-33-35_001_091714.bin", "mod time(min)"=58229553.583333336, "file format"=enum."binary", "power(V)"=2.1, "Magn Field(T) "=0.0}, {"temperature"=84.704, "temperature str"="84.70400", "file path"=path "D:/Data/Ultrasound/LSCO/LSCO22__130814c/5_Cooling_2nd_try/September_2014/091714/84.70400K_500_2500_2.10000V_0.00000T_Sep17-2014__00-34-55_001_091714.bin", "last mod"=timestamp(3493773295 s since 1904-01-01), "file name str"="D:\\Data\\Ultrasound\\LSCO\\LSCO22__130814c\\5_Cooling_2nd_try\\September_2014\\091714\\84.70400K_500_2500_2.10000V_0.00000T_Sep17-2014__00-34-55_001_091714.bin", "mod time(min)"=58229554.916666664, "file format"=enum."binary", "power(V)"=2.1, "Magn Field(T) "=0.0}, {"temperature"=84.597, "temperature str"="84.59700", "file path"=path "D:/Data/Ultrasound/LSCO/LSCO22__130814c/5_Cooling_2nd_try/September_2014/091714/84.59700K_500_2500_2.10000V_0.00000T_Sep17-2014__00-36-14_001_091714.bin", "last mod"=timestamp(3493773374 s since 1904-01-01), "file name str"="D:\\Data\\Ultrasound\\LSCO\\LSCO22__130814c\\5_Cooling_2nd_try\\September_2014\\091714\\84.59700K_500_2500_2.10000V_0.00000T_Sep17-2014__00-36-14_001_091714.bin", "mod time(min)"=58229556.233333334, "file format"=enum."binary", "power(V)"=2.1, "Magn Field(T) "=0.0}, {"temperature"=84.501, "temperature str"="84.50100", "file path"=path "D:/Data/Ultrasound/LSCO/LSCO22__130814c/5_Cooling_2nd_try/September_2014/091714/84.50100K_500_2500_2.10000V_0.00000T_Sep17-2014__00-37-33_001_091714.bin", "last mod"=timestamp(3493773453 s since 1904-01-01), "file name str"="D:\\Data\\Ultrasound\\LSCO\\LSCO22__130814c\\5_Cooling_2nd_try\\September_2014\\091714\\84.50100K_500_2500_2.10000V_0.00000T_Sep17-2014__00-37-33_001_091714.bin", "mod time(min)"=58229557.55, "file format"=enum."binary", "power(V)"=2.1, "Magn Field(T) "=0.0}, {"temperature"=84.397, "temperature str"="84.39700", "file path"=path "D:/Data/Ultrasound/LSCO/LSCO22__130814c/5_Cooling_2nd_try/September_2014/091714/84.39700K_500_2500_2.10000V_0.00000T_Sep17-2014__00-38-53_001_091714.bin", "last mod"=timestamp(3493773533 s since 1904-01-01), "file name str"="D:\\Data\\Ultrasound\\LSCO\\LSCO22__130814c\\5_Cooling_2nd_try\\September_2014\\091714\\84.39700K_500_2500_2.10000V_0.00000T_Sep17-2014__00-38-53_001_091714.bin", "mod time(min)"=58229558.88333333, "file format"=enum."binary", "power(V)"=2.1, "Magn Field(T) "=0.0}, {"temperature"=84.293, "temperature str"="84.29300", "file path"=path "D:/Data/Ultrasound/LSCO/LSCO22__130814c/5_Cooling_2nd_try/September_2014/091714/84.29300K_500_2500_2.10000V_0.00000T_Sep17-2014__00-40-12_001_091714.bin", "last mod"=timestamp(3493773612 s since 1904-01-01), "file name str"="D:\\Data\\Ultrasound\\LSCO\\LSCO22__130814c\\5_Cooling_2nd_try\\September_2014\\091714\\84.29300K_500_2500_2.10000V_0.00000T_Sep17-2014__00-40-12_001_091714.bin", "mod time(min)"=58229560.2, "file format"=enum."binary", "power(V)"=2.1, "Magn Field(T) "=0.0}, {"temperature"=84.193, "temperature str"="84.19300", "file path"=path "D:/Data/Ultrasound/LSCO/LSCO22__130814c/5_Cooling_2nd_try/September_2014/091714/84.19300K_500_2500_2.10000V_0.00000T_Sep17-2014__00-41-31_001_091714.bin", "last mod"=timestamp(3493773691 s since 1904-01-01), "file name str"="D:\\Data\\Ultrasound\\LSCO\\LSCO22__130814c\\5_Cooling_2nd_try\\September_2014\\091714\\84.19300K_500_2500_2.10000V_0.00000T_Sep17-2014__00-41-31_001_091714.bin", "mod time(min)"=58229561.516666666, "file format"=enum."binary", "power(V)"=2.1, "Magn Field(T) "=0.0}, {"temperature"=84.09, "temperature str"="84.09000", "file path"=path "D:/Data/Ultrasound/LSCO/LSCO22__130814c/5_Cooling_2nd_try/September_2014/091714/84.09000K_500_2500_2.10000V_0.00000T_Sep17-2014__00-42-51_001_091714.bin", "last mod"=timestamp(3493773771 s since 1904-01-01), "file name str"="D:\\Data\\Ultrasound\\LSCO\\LSCO22__130814c\\5_Cooling_2nd_try\\September_2014\\091714\\84.09000K_500_2500_2.10000V_0.00000T_Sep17-2014__00-42-51_001_091714.bin", "mod time(min)"=58229562.85, "file format"=enum."binary", "power(V)"=2.1, "Magn Field(T) "=0.0}, {"temperature"=83.993, "temperature str"="83.99300", "file path"=path "D:/Data/Ultrasound/LSCO/LSCO22__130814c/5_Cooling_2nd_try/September_2014/091714/83.99300K_500_2500_2.10000V_0.00000T_Sep17-2014__00-44-10_001_091714.bin", "last mod"=timestamp(3493773850 s since 1904-01-01), "file name str"="D:\\Data\\Ultrasound\\LSCO\\LSCO22__130814c\\5_Cooling_2nd_try\\September_2014\\091714\\83.99300K_500_2500_2.10000V_0.00000T_Sep17-2014__00-44-10_001_091714.bin", "mod time(min)"=58229564.166666664, "file format"=enum."binary", "power(V)"=2.1, "Magn Field(T) "=0.0}, {"temperature"=83.89, "temperature str"="83.89000", "file path"=path "D:/Data/Ultrasound/LSCO/LSCO22__130814c/5_Cooling_2nd_try/September_2014/091714/83.89000K_500_2500_2.10000V_0.00000T_Sep17-2014__00-45-30_001_091714.bin", "last mod"=timestamp(3493773930 s since 1904-01-01), "file name str"="D:\\Data\\Ultrasound\\LSCO\\LSCO22__130814c\\5_Cooling_2nd_try\\September_2014\\091714\\83.89000K_500_2500_2.10000V_0.00000T_Sep17-2014__00-45-30_001_091714.bin", "mod time(min)"=58229565.5, "file format"=enum."binary", "power(V)"=2.1, "Magn Field(T) "=0.0}, {"temperature"=83.79, "temperature str"="83.79000", "file path"=path "D:/Data/Ultrasound/LSCO/LSCO22__130814c/5_Cooling_2nd_try/September_2014/091714/83.79000K_500_2500_2.10000V_0.00000T_Sep17-2014__00-46-49_001_091714.bin", "last mod"=timestamp(3493774009 s since 1904-01-01), "file name str"="D:\\Data\\Ultrasound\\LSCO\\LSCO22__130814c\\5_Cooling_2nd_try\\September_2014\\091714\\83.79000K_500_2500_2.10000V_0.00000T_Sep17-2014__00-46-49_001_091714.bin", "mod time(min)"=58229566.81666667, "file format"=enum."binary", "power(V)"=2.1, "Magn Field(T) "=0.0}, {"temperature"=83.692, "temperature str"="83.69200", "file path"=path "D:/Data/Ultrasound/LSCO/LSCO22__130814c/5_Cooling_2nd_try/September_2014/091714/83.69200K_500_2500_2.10000V_0.00000T_Sep17-2014__00-48-08_001_091714.bin", "last mod"=timestamp(3493774088 s since 1904-01-01), "file name str"="D:\\Data\\Ultrasound\\LSCO\\LSCO22__130814c\\5_Cooling_2nd_try\\September_2014\\091714\\83.69200K_500_2500_2.10000V_0.00000T_Sep17-2014__00-48-08_001_091714.bin", "mod time(min)"=58229568.13333333, "file format"=enum."binary", "power(V)"=2.1, "Magn Field(T) "=0.0}, {"temperature"=83.591, "temperature str"="83.59100", "file path"=path "D:/Data/Ultrasound/LSCO/LSCO22__130814c/5_Cooling_2nd_try/September_2014/091714/83.59100K_500_2500_2.10000V_0.00000T_Sep17-2014__00-49-28_001_091714.bin", "last mod"=timestamp(3493774168 s since 1904-01-01), "file name str"="D:\\Data\\Ultrasound\\LSCO\\LSCO22__130814c\\5_Cooling_2nd_try\\September_2014\\091714\\83.59100K_500_2500_2.10000V_0.00000T_Sep17-2014__00-49-28_001_091714.bin", "mod time(min)"=58229569.46666667, "file format"=enum."binary", "power(V)"=2.1, "Magn Field(T) "=0.0}, {"temperature"=83.495, "temperature str"="83.49500", "file path"=path "D:/Data/Ultrasound/LSCO/LSCO22
